vi "ConfigMessageMetadata.vi"(7 "ConcreteMessage":refnum<class "ConcreteMessage.lvclass">, 9 "TellOrigin":T2, 10 "Lifetime":T1, 11 "ActorAlias":string) -> (5 "ConcreteMessage":refnum<class "ConcreteMessage.lvclass">)   [LabVIEW 2020, in "_Template.lvlib" / "MessageTemplate.lvlib" / "{{Name}}.lvlib" / "ConcreteMessage.lvclass"]
uses:
  ConcreteMessage.lvclass
  ConcreteMessage.lvclass/ConcreteMessage.ctl
  jettl/jettl/jettl.lvlib
  jettl/jettl/Lifetime.ctl
  jettl/jettl/TellOrigin.ctl
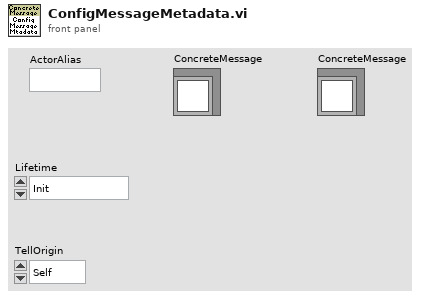
[diagram p1: front panel]
types:
  T1 = typedef "jettl.lvlib/Lifetime.ctl" = enum16{"Init", "Spawn", "Setup", "TeardownBeforeRunning", "Running", "StopCalled", "StoppingWithComponents", "StoppingNoComponents", "TeardownAfterRunning", "Stopped"}
  T2 = typedef "jettl.lvlib/TellOrigin.ctl" = enum16{"Self", "Mediator", "Component"}
  T3 = typedef "jettl.lvlib/MessageMetadata.ctl" = cluster{"ActorAlias":string, "Lifetime":T1, "TellOrigin":T2, "AbsoluteTime":timestamp, "RelativeTime":dbl}
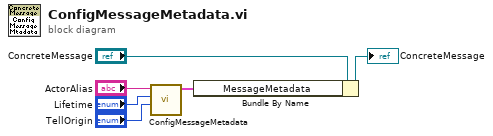
[diagram p0: block diagram]
diagram:
  n1 = call "ConfigMessageMetadata.vi"("TellOrigin"="TellOrigin", "Lifetime"="Lifetime", "ActorAlias"="ActorAlias") -> ("MessageMetadata"=w4:T3)  [unwired: 8 in]
  n2 = Bundle By Name(cluster="ConcreteMessage", "MessageMetadata"=w4) -> (→"ConcreteMessage":refnum<class "ConcreteMessage.lvclass">)
